vi "Pick Top 3.vi"(0 "Min Pts":i32=3, 1 "Histogram Graph":T1) -> (2 "spacing":dbl, 4 "Top 3":dbl[](array[numeric]))   [LabVIEW 2013]
doc: "Return X positions of up to three bins with the highest number of particles, and spacing between the bins."
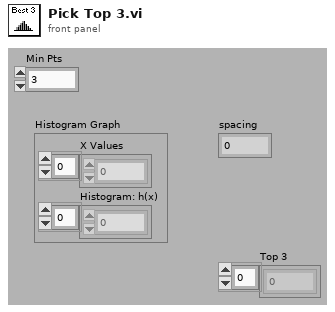
[diagram p1: front panel]
types:
  T1 = cluster{"X Values":dbl[], "Histogram: h(x)":i32[]}
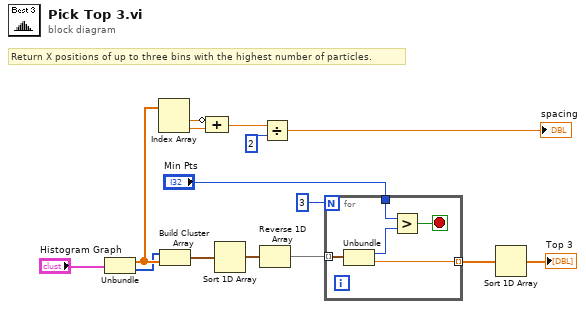
[diagram p0: block diagram]
diagram:
  # "Return X positions of up to three bins with the highest number of particles."
  n1 = Unbundle("Histogram Graph") -> ("X Values"=w8:dbl[], "Histogram: h(x)"=w2:i32[])
  n2 = Index Array(array=w8) -> (element #1=w9:dbl, element #2=w10:dbl)  [unwired: 2 in]
  n3 = Build Cluster Array(w2, w8) -> (w3:cluster{i32, dbl}[])
  n4 = Compound Arithmetic op=ADD(invert w9, w10) -> (w11:dbl)
  n5 = Sort 1D Array(array=w3) -> (sorted array=w4:cluster{i32, dbl}[])
  n6 = Reverse 1D Array(array=w4) -> (reversed array=w5:cluster{i32, dbl}[])
  n7 = Divide(x=w11, y=2) -> (x/y=→"spacing":dbl)
  n8 = for {
    N: 3 -> [_]
    tunnel: w5 -> [w20] mode=indexing
    tunnel: [w19] -> w7 mode=indexing
    tunnel: "Min Pts" -> [w16]
    stop <- w18 stop-if-true
    n9 = Unbundle(w20) -> (w17:i32, w19:dbl)
    n10 = Greater?(x=w16, y=w17) -> (0:w18:bool)
  }
  n11 = Sort 1D Array(array=w7) -> (sorted array=→"Top 3":dbl[])
